vi "MQTT_Read_Subscribed_Topics.vi"(8 "error in (no error)":errorcluster) -> (0 "error out":errorcluster)   [LabVIEW 2019, in "MQTT_Functions.lvlib"]
doc: "A basic example that reads topics that the client subcribed to. \n\n© 2015 - daq.io, LLC - Peter Adelhardt"
uses:
  MQTT_Functions.lvlib
  Controls/QoS.ctl
  Controls/Connect_Flags.ctl
  Controls/Retain_Flag.ctl
  Controls/DUP_Flag.ctl
  Controls/Connection_Return_Codes.ctl
panel:
  out "Connection Status":T1=enum."Connection refused: not authorized"
  in  "Exit":bool
  in  "MQTT Broker":cluster{"address (IP)":string, "port":u16}={"address (IP)"="broker.hivemq.com", "port"=1883}
  out "Message IDs":u16[](array[numeric]) format="%x"
  out "Topics":string[](array[string])
  out "Messages":string[](array[string])
  in  "Client ID":string="LVSubscribeClient"
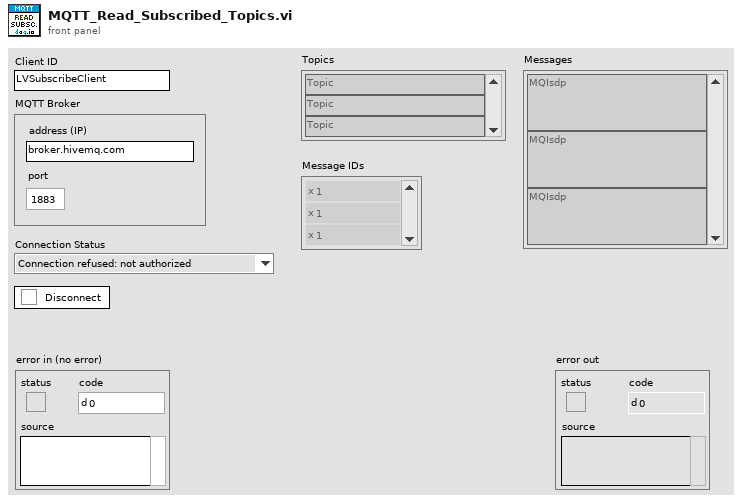
[diagram p1: front panel]
types:
  T1 = typedef "MQTT_Functions.lvlib/Connection_Return_Codes.ctl" = enum16{"Connection accepted", "Connection refused: unacceptable protocol version", "Connection refused: identifier rejected", "Connection refused: Server unavailable", "Connection refused: bad user name or password", "Connection refused: not authorized"}
  T2 = typedef "MQTT_Functions.lvlib/QoS.ctl" = enum8{"At most once", "At least once", "Exactly once", "Reserved"}
  T3 = typedef "MQTT_Functions.lvlib/DUP_Flag.ctl" = bool
  T4 = typedef "MQTT_Functions.lvlib/Retain_Flag.ctl" = bool
  T5 = cluster{"QoS":T2, "DUP":T3, "Retain":T4, "Keep Alive (sec)":u16}
  T6 = typedef "MQTT_Functions.lvlib/Connect_Flags.ctl" = cluster{"user name":bool, "password":bool, "will retain":bool, "will flag":bool, "clean session":bool, "reserved":bool, "will QoS":T2}
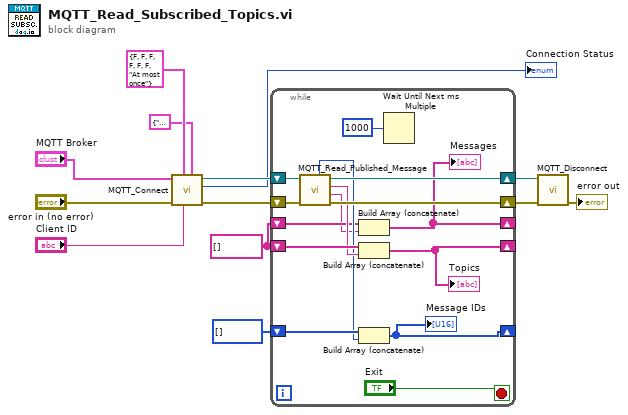
[diagram p0: block diagram]
diagram:
  w6 = string[] []
  n1 = call "MQTT_Connect.vi"("Connect Meta"=T5 {"QoS"=enum."At most once", "DUP"=FALSE, "Retain"=FALSE, "Keep Alive (sec)"=60}, "Client ID"="Client ID", "Connect Flags"=T6 {"user name"=FALSE, "password"=FALSE, "will retain"=FALSE, "will flag"=FALSE, "clean session"=FALSE, "reserved"=FALSE, "will QoS"=enum."At most once"}, "error in (no error)"="error in (no error)", "MQTT Broker Details"="MQTT Broker") -> ("error out"=w1:errorcluster, "Connection Status"=→"Connection Status":T1, "connection ID out"=w3:refnum<k5>)  [unwired: 4 in]
  n2 = while {
    shift-right: [w23] -> w8
    shift-left: w1 -> [w25]
    shift-right: [w14] -> _
    shift-left: u16[] [] -> [w20]
    shift-right: [w15] -> _
    shift-left: w6 -> [w18]
    shift-right: [w16] -> _
    shift-left: w6 -> [w22]
    shift-right: [w24] -> w9
    shift-left: w3 -> [w26]
    stop <- "Exit" stop-if-true
    n3 = call "MQTT_Read_Published_Message.vi"("error in (no error)"=w25, "connection ID"=w26) -> ("error out"=w23:errorcluster, "Message"=w17:string, "Topic Name"=w21:string, "connection ID out"=w24:refnum<k5>, "Message ID"=w19:u16)  [unwired: 4 in, 1 out]
    n4 = Build Array (concatenate)(w18, w17) -> (w15:string[])
    "Messages" <- w15
    n5 = Build Array (concatenate)(w22, w21) -> (w16:string[])
    "Topics" <- w16
    n6 = Build Array (concatenate)(w20, w19) -> (w14:u16[])
    "Message IDs" <- w14
    n7 = Wait Until Next ms Multiple(millisecond multiple=u32 1000) -> ()  [unwired: 1 out]
  }
  n8 = call "MQTT_Disconnect.vi"("error in (no error)"=w8, "connection ID"=w9) -> ("error out"=→"error out":errorcluster)  [unwired: 9 in]
